vi "BK.vi"(8 "error in (no error)":errorcluster, 11 "NPad2 in":refnum<class "NPad2.lvclass">) -> (0 "error out":errorcluster, 3 "NPad2 out":refnum<class "NPad2.lvclass">)   [LabVIEW 2020, in "NPad2.lvlib" / "NPad2.lvclass"]
uses:
  NPad2.lvclass
  NPad2.lvclass/NPad2.ctl
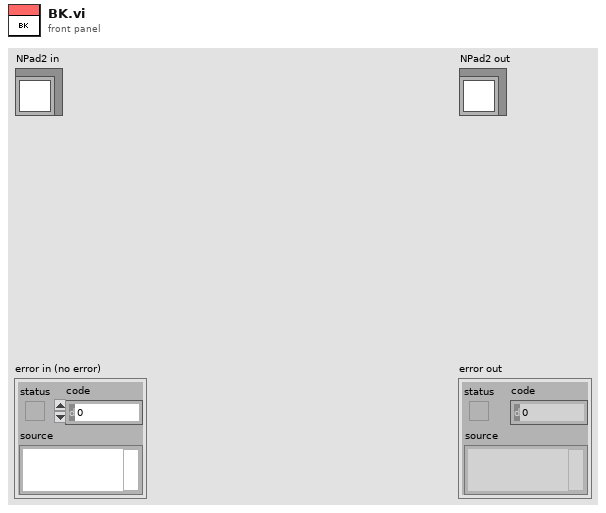
[diagram p1: front panel]
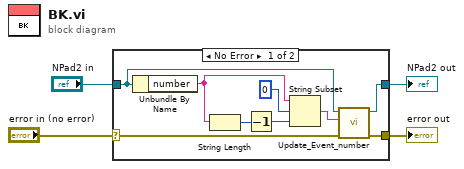
[diagram p0: block diagram]
diagram:
  n1 = case shown="No Error" "error in (no error)" {
    selector: "error in (no error)" -> [w6 w15]
    tunnel: [w5 w15] -> w3
    tunnel: [w7 w14] -> w1
    tunnel: "NPad2 in" -> [w8 w14]
    frame No Error {
      n2 = Unbundle By Name(w8) -> ("number"=w13:string)
      n3 = String Length(string=w13) -> (length=w11:i32)
      n4 = Decrement(x=w11) -> (x-1=w10:i32)
      n5 = String Subset(string=w13, offset (0)=0, length (rest)=w10) -> (substring=w9:string)
      n6 = call "Update_Event_number.vi"("error in (no error)"=w6, "number"=w9, "NPad2 in"=w8) -> ("error out"=w5:errorcluster, "NPad2 out"=w7:refnum<class "NPad2.lvclass">)  [unwired: 7 in]
    }
    frame Error {
    }
  }
  "error out" <- w3
  "NPad2 out" <- w1
